vi "getStatus.vi"(8 "error in (no error)":errorcluster, 10 "SpectrographClientCommunicator in":refnum<class "SpectrographClientCommunicator.lvclass">, 11 "SpectrographHeartbeat in":refnum<class "SpectrographHeartbeat.lvclass">) -> (0 "error out":errorcluster, 2 "SpectrographClientCommunicator out":refnum<class "SpectrographClientCommunicator.lvclass">, 3 "SpectrographHeartbeat out":refnum<class "SpectrographHeartbeat.lvclass">, 4 "timeout?":bool, 5 "newValue":bool)   [LabVIEW 2016, in "SpectrographHeartbeat.lvclass"]
uses:
  SpectrographHeartbeat.lvclass
  SpectrographClientCommunicator/SpectrographClientCommunicator.lvclass
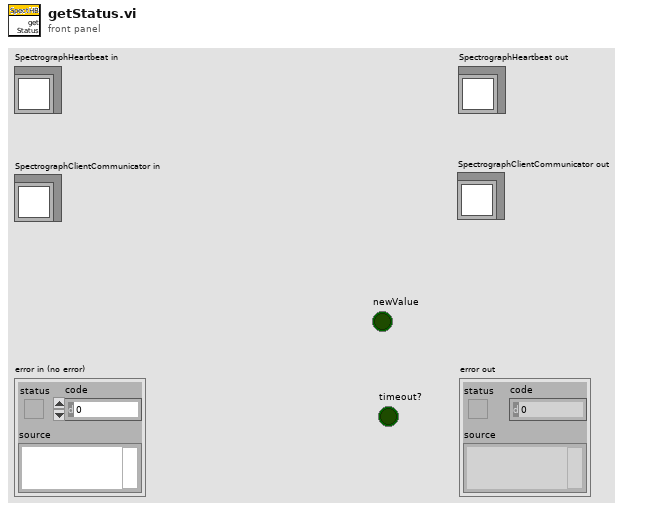
[diagram p1: front panel]
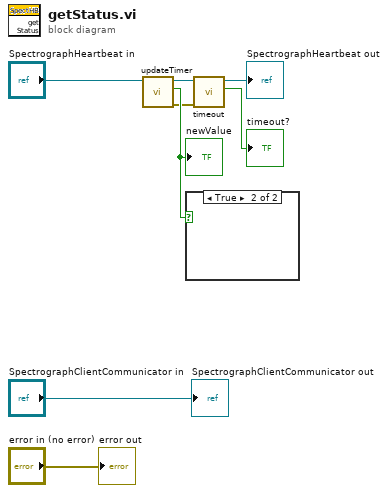
[diagram p0: block diagram]
diagram:
  n1 = call "updateTimer.vi"("SpectrographHeartbeat in"="SpectrographHeartbeat in") -> ("error out"=w3:errorcluster, "getStatus?"=w6:bool, "SpectrographHeartbeat out"=w2:refnum<class "SpectrographHeartbeat.lvclass">)  [unwired: 8 in]
  "newValue" <- w6
  n2 = case shown="True" w6 {
    frame False {
    }
    frame True {
    }
  }
  n3 = call "timeout.vi"("error in (no error)"=w3, "SpectrographHeartbeat in"=w2) -> ("timeout?"=→"timeout?":bool, "SpectrographHeartbeat out"=→"SpectrographHeartbeat out":refnum<class "SpectrographHeartbeat.lvclass">)  [unwired: 7 in, 1 out]
  "error out" <- "error in (no error)"
  "SpectrographClientCommunicator out" <- "SpectrographClientCommunicator in"
